vi "A 正面 处理函数2.vi"(7 "error in":errorcluster) -> (27 "error out":errorcluster)   [LabVIEW 2017]
uses:
  <vilib>/vision/Measure.llb/Edge Options.ctl
  <vilib>/vision/Measure.llb/Edge Polarity.ctl
  <vilib>/vision/Contour.llb/IMAQ Connect Range Setting.ctl
  <vilib>/vision/Contour.llb/IMAQ Contour Curve Extraction.ctl
  <vilib>/vision/Pattern Matching.llb/IMAQ Match Range Setting.ctl
  <vilib>/vision/NI_Vision_Development_Module.lvlib
panel:
  out "Image Out":T1(plugin-control)
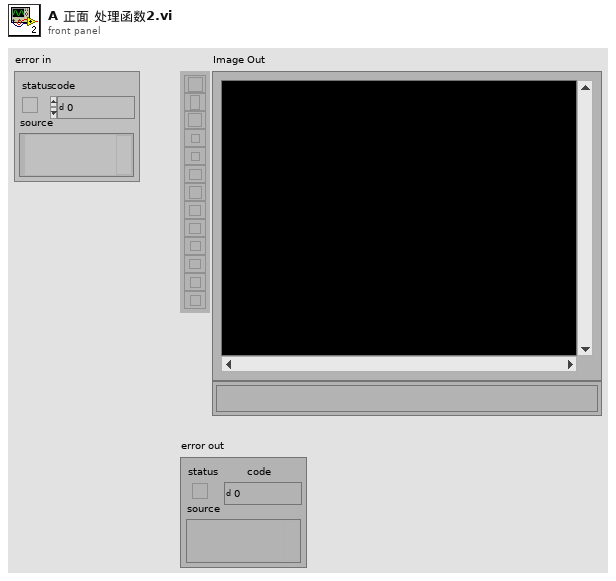
[diagram p1: front panel]
types:
  T1 = typedef "IMAQ Image.ctl" = refnum<image>
  T2 = typedef "IMAQ Match Range Setting.ctl" = cluster{"Match Constraints":u32, "Min":dbl, "Max":dbl}
  T3 = cluster{"Setup Data Item":u16, "Item Value":dbl}[]
  T4 = typedef "IMAQ Contour Curve Extraction.ctl" = cluster{"Extraction Mode":u32, "Edge Threshold":i32, "Edge Filter Size":u32, "Min Length":i32, "Search Step Size":i32, "Max Endpoint Gap":i32, "Subpixel":bool}
  T5 = cluster{"Rotation":bool, "Scale":bool, "Occlusion":bool}
  T6 = typedef "IMAQ Connect Range Setting.ctl" = cluster{"Match Constraints":u32, "Min":dbl, "Max":dbl}
  T7 = enum16{"Closest To Search Start", "Maximum Length", "Strongest Mean Gradient Change"}
  T8 = enum16{"Rect Left To Right", "Rect Right To Left", "Rect Top To Bottom", "Rect Bottom To Top", "Annulus Inner To Outer", "Annulus Outer To Inner", "Annulus Start Angle To End Angle", "Annulus End Angle To Start Angle"}
  T9 = cluster{"Overlay?":bool, "Color":u32, "Width":u32, "Maintain Width?":bool}
  T10 = cluster{"Global Rectangle":i32[], "Contours":cluster{"ID":enum32{"External", "Internal"}, "Type":u32, "Coordinates":i32[]}[]}
  T11 = cluster{"Origin":cluster{"X":sgl, "Y":sgl}, "Angle (deg)":sgl, "Axis Reference":u32}
  T12 = enum16{"Reset", "Update Coordinate System", "Get Coordinate System"}
  T13 = enum16{"Horizontal Motion", "Vertical Motion", "Horizontal and Vertical Motion", "Horizontal, Vertical and Angular Motion"}
  T14 = typedef "Edge Options.ctl" = cluster{"Edge Polarity":T15, "Kernel Size":u32, "Width":u32, "Minimum Edge Strength":sgl, "Interpolation Type":enum32{"Zero Order", "Bilinear", "Quadratic", "Cubic", "Bilinear Fixed"}, "Data Processing Method":enum32{"Average", "Median"}}
  T15 = typedef "Edge Polarity.ctl" = u32
  T16 = cluster{"Search  Direction":u32, "Edge Options":T14, "Show Search Area":bool, "Show Search Lines":bool, "Show Edges Found":bool, "Show Result":bool, "Search Area Color":u32, "Search Lines Color":u32, "Edge Locations Color":u32, "Result Color":u32, "Overlay Group Name":string}
  T17 = cluster{"Process":enum16{"Get First Edge", "Get First + Last Edge", "Get All Edges", "Get Best Edge"}, "Step Size":i32, "Max Pixel Radius":i32}
  T18 = typedef "Image Type" = u32
  T19 = cluster{"Center (Pixels)":cluster{"X":sgl, "Y":sgl}, "Radius (Pixels)":dbl, "Center (Real-World)":cluster{"X":sgl, "Y":sgl}, "Radius (Real-World)":dbl, "Roundness (Real-World)":dbl, "Average Strength":dbl, "Average SNR (dB)":dbl}
  T20 = typedef "IMAQ Coordinate System" = cluster{"Reference System":cluster{"Origin":cluster{"X":sgl, "Y":sgl}, "Angle (deg)":sgl, "Axis Reference":u32}, "Measurement System":cluster{"Origin":cluster{"X":sgl, "Y":sgl}, "Angle (deg)":sgl, "Axis Reference":u32}}
  T21 = typedef "ROI Descriptor" = cluster{"Global Rectangle":i32[], "Contours":cluster{"ID":enum32{"External", "Internal"}, "Type":u32, "Coordinates":i32[]}[]}
  T22 = cluster{"Target Point":cluster{"X":dbl, "Y":dbl}, "Template Point":cluster{"X":dbl, "Y":dbl}, "Distance":dbl}[]
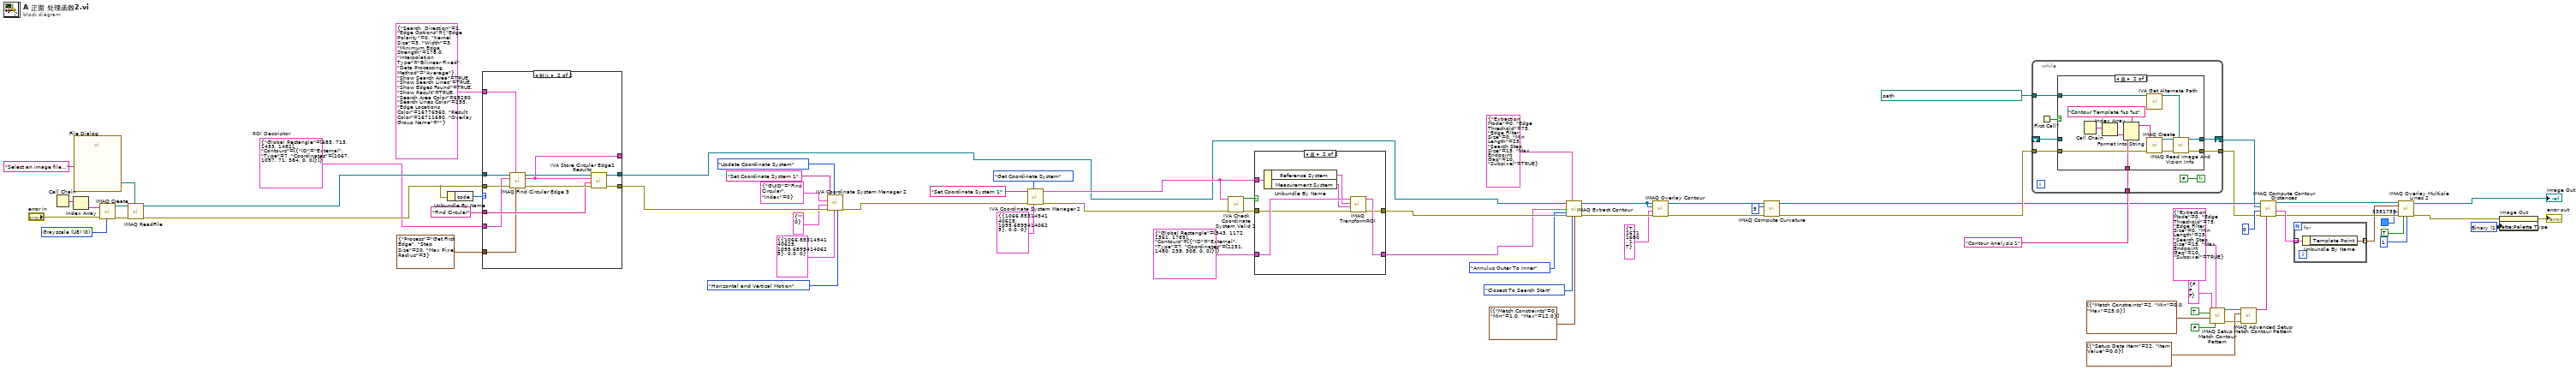
[diagram p0: block diagram]
diagram:
  w1 = u32 1 items=["Grayscale", "Binary", "Gradient", "Rainbow", "Temperature", "User Defined", "Binary 16 Bit", "Gradient 16 Bit", "Rainbow 16 Bit", "Temperature 16 Bit", "User Defined 16 Bit"] ("Palette Type")
  w59 = T10 {"Global Rectangle"=[683, 713, 1453, 1482], "Contours"=[{"ID"=enum."External", "Type"=7, "Coordinates"=[1067, 1097, 71, 384, 0, 0]}]}  # ROI Descriptor
  w63 = T18 0 items=["Grayscale (U8)", "Grayscale (I16)", "Grayscale (SGL)", "Complex (CSG)", "RGB (U32)", "HSL (U32)", "RGB (U64)", "Grayscale (U16)"] ("Image Type")
  n1 = Call Chain() -> (call chain=w67:string[])
  n2 = Index Array(array=w67) -> (element=w66:string)  [unwired: 1 in]
  n3 = call "File Dialog"("prompt"="Select an image file...") -> ("selected path"=w64:path)  [unwired: 6 in, 8 out]
  n4 = call "IMAQ Create"("Image Name"=w66, "Image Type"=w63, "error in (no error)"="error in") -> ("New Image"=w70:T1, "error out"=w69:errorcluster)  [unwired: 1 in, 1 out]
  n5 = call "IMAQ ReadFile"("File Path"=w64, "error in (no error)"=w69, "Image"=w70) -> ("error out"=w71:errorcluster, "Image Out"=w62:T1)  [unwired: 2 in, 5 out]
  n6 = Unbundle By Name(w71) -> ("code"=w58:i32)
  n7 = case "条件结构" shown="默认" w58 {
    tunnel: T16 {"Search  Direction"=1, "Edge Options"={"Edge Polarity"=0, "Kernel Size"=3, "Width"=3, "Minimum Edge Strength"=178.0, "Interpolation Type"=enum."Bilinear Fixed", "Data Processing Method"=enum."Average"}, "Show Search Area"=TRUE, "Show Search Lines"=TRUE, "Show Edges Found"=TRUE, "Show Result"=TRUE, "Search Area Color"=65280, "Search Lines Color"=255, "Edge Locations Color"=16776960, "Result Color"=16711680, "Overlay Group Name"=""} ("Options") -> [_ w73]
    tunnel: w62 -> [w72 w83]
    tunnel: w71 -> [_ w82]
    tunnel: [_ w80] -> w61
    tunnel: [w72 w78] -> w39
    tunnel: "Find Circular" ("Step Name") -> [_ w77]
    tunnel: w59 -> [_ w76]
    tunnel: T17 {"Process"=enum."Get First Edge", "Step Size"=20, "Max Pixel Radius"=3} ("Circle Fit Options") -> [_ w75]
    tunnel: [_ w74] -> _
    frame -1074396199, -1074396198 {
      # "Discard Coordinate System Error"
    }
    frame Default {
      n8 = call "IMAQ Find Circular Edge 3"("Circle Fit Options"=w75, "Options"=w73, "error in (no error)"=w82, "ROI Descriptor"=w76, "Image"=w83) -> ("error out"=w81:errorcluster, "Fitted Circle"=w74:T19, "Image Out"=w79:T1)  [unwired: 2 in, 2 out]
      n9 = call <vilib>:"IVA Store Circular Edge2 Results.vi"("error in (no error)"=w81, "Step Name"=w77, "Fitted Circle"=w74, "Image in"=w79) -> ("error out"=w80:errorcluster, "Image dup"=w78:T1)  [unwired: 2 in, 4 out]
    }
  }
  n10 = call <vilib>:"IVA Coordinate System Manager 2.vi"("Mode"=T13."Horizontal and Vertical Motion", "Reference System"=T11 {"Origin"={"X"=1066.8531, "Y"=1095.69}, "Angle (deg)"=0.0, "Axis Reference"=0}, "Function"=T12."Update Coordinate System", "error in (no error)"=w61, "Angle ID"=cluster{"GUID":string, "Index":i32} {"GUID"="", "Index"=0}, "Origin ID"=cluster{"GUID":string, "Index":i32} {"GUID"="Find Circular", "Index"=0}, "Coordinate System Name"="Set Coordinate System 1") -> ("error out"=w49:errorcluster)  [unwired: 4 out]
  n11 = call <vilib>:"IVA Coordinate System Manager 2.vi"("Reference System"=T11 {"Origin"={"X"=1066.8531, "Y"=1095.69}, "Angle (deg)"=0.0, "Axis Reference"=0}, "Function"=T12."Get Coordinate System", "error in (no error)"=w49, "Coordinate System Name"="Set Coordinate System 1") -> ("error out"=w46:errorcluster, "Coordinate System Out"=w42:T20)  [unwired: 3 in, 3 out]
  n12 = call <vilib>:"IVA Check Coordinate System Valid 2.vi"("error in (no error)"=w46, "Coordinate System"=w42) -> ("error out"=w40:errorcluster, "Valid?"=w41:bool)  [unwired: 8 out]
  n13 = case "条件结构" shown="真" w41 {
    tunnel: T10 {"Global Rectangle"=[943, 1172, 1561, 1789], "Contours"=[{"ID"=enum."External", "Type"=7, "Coordinates"=[1251, 1480, 238, 308, 0, 0]}]} ("ROI Descriptor") -> [w85 w92]
    tunnel: [w85 w89] -> w35
    tunnel: [w84 w88] -> w43
    tunnel: w42 -> [_ w87]
    tunnel: w40 -> [w84 w86]
    frame False {
    }
    frame True {
      n14 = Unbundle By Name(w87) -> ("Reference System"=w91:T11, "Measurement System"=w90:T11)
      n15 = call "IMAQ TransformROI"("error in (no error)"=w86, "New Reference"=w90, "Base Reference"=w91, "ROI Descriptor"=w92) -> ("error out"=w88:errorcluster, "ROI Descriptor out"=w89:T21)  [unwired: 6 out]
    }
  }
  n16 = call "IMAQ Extract Contour"("Source Image"=w39, "Curve Extraction"=T4 {"Extraction Mode"=0, "Edge Threshold"=75, "Edge Filter Size"=0, "Min Length"=25, "Search Step Size"=15, "Max Endpoint Gap"=10, "Subpixel"=TRUE}, "ROI Descriptor"=w35, "Search Direction"=T8."Annulus Outer To Inner", "error in (no error)"=w43, "Contour Selection"=T7."Closest To Search Start", "Curve Connection"=T6[] [{"Match Constraints"=0, "Min"=1.0, "Max"=12.0}]) -> ("Source Image Out"=w31:T1, "error out"=w38:errorcluster)  [unwired: 1 in, 6 out]
  n17 = call "IMAQ Overlay Contour"("error in (no error)"=w38, "Contour Points Settings"=T9 {"Overlay?"=TRUE, "Color"=16711680, "Width"=1, "Maintain Width?"=TRUE}, "Contour Image"=w31, "Image"=w31) -> ("error out"=w36:errorcluster, "Image Out"=w29:T1)  [unwired: 2 in, 4 out]
  n18 = call "IMAQ Compute Curvature"("error in (no error)"=w36, "Kernel Width"=u32 5, "Contour Image"=w29) -> ("error out"=w28:errorcluster, "Contour Image Out (dup)"=w23:T1)  [unwired: 1 in, 6 out]
  n19 = while "While循环" {
    tunnel: path "C:/Users/hedongpo/Desktop/吕亚/Temp3.png" ("Template File Path") -> [w100]
    tunnel: "Contour Analysis 1" ("Step Name") -> [w98]
    shift-right: [w96] -> w22
    shift-left: _ -> [w97]
    tunnel: w28 -> [w95]
    tunnel: [w94] -> w21
    stop <- FALSE continue-if-true
    n20 = First Call?() -> (First Call?: T/F=w99:bool)
    n21 = case "条件结构" shown="真" w99 {
      tunnel: [w102 w104] -> w96
      tunnel: w97 -> [w102 _]
      tunnel: [w101 w103] -> w94
      tunnel: w95 -> [w101 w109]
      tunnel: w100 -> [_ w114]
      tunnel: w98 -> [_ w105]
      frame False {
      }
      frame True {
        n22 = Call Chain() -> (call chain=w111:string[])
        n23 = Index Array(array=w111) -> (element=w110:string)  [unwired: 1 in]
        n24 = Format Into String(format string="Contour Template %s %s" ("Image Name"), w110, w105) -> (resulting string=w113:string)  [unwired: 2 in, 1 out]
        n25 = call <vilib>:"IVA Get Alternate Path.vi"("Path In"=w114) -> ("Path Out"=w106:path)  [unwired: 10 out]
        n26 = call "IMAQ Create"("Image Name"=w113, "error in (no error)"=w109) -> ("New Image"=w108:T1, "error out"=w107:errorcluster)  [unwired: 2 in, 1 out]
        n27 = call "IMAQ Read Image And Vision Info"("File Path"=w106, "error in (no error)"=w107, "Image"=w108) -> ("error out"=w103:errorcluster, "Image Out"=w104:T1)  [unwired: 1 in, 6 out]
      }
    }
  }
  n28 = call "IMAQ Setup Match Contour Pattern"("Use Learn Curve Extraction"=FALSE, "Curve Extraction"=T4 {"Extraction Mode"=0, "Edge Threshold"=75, "Edge Filter Size"=0, "Min Length"=25, "Search Step Size"=15, "Max Endpoint Gap"=10, "Subpixel"=TRUE} ("Curve Extraction 2"), "Range Settings"=T2[] [{"Match Constraints"=2, "Min"=0.0, "Max"=25.0}], "Subpixel Accuracy"=TRUE, "Match Mode"=T5 {"Rotation"=FALSE, "Scale"=FALSE, "Occlusion"=FALSE}) -> ("error out"=w4:errorcluster, "Match Contour Pattern Setup Data"=w8:string)  [unwired: 1 in, 4 out]
  n29 = call "IMAQ Advanced Setup Match Contour Pattern"("Match Contour Pattern Setup Data In"=w8, "Advanced Contour Match Options"=T3 [{"Setup Data Item"=22, "Item Value"=0.0}], "error in (no error)"=w4) -> ("Match Contour Pattern Setup Data Out"=w7:string)  [unwired: 7 out]
  n30 = call "IMAQ Compute Contour Distances"("Match Contour Pattern Setup Data"=w7, "error in (no error)"=w21, "Smoothing Kernel"=u32 0, "Template Contour Image"=w22, "Target Contour Image"=w23) -> ("error out"=w15:errorcluster, "Distances"=w17:T22, "Target Contour Image Out (dup)"=w16:T1)  [unwired: 4 out]
  n31 = for "For循环" {
    tunnel: w17 -> [w116] mode=indexing
    tunnel: [w115] -> w14 mode=indexing
    n32 = Unbundle By Name(w116) -> ("Template Point"=w115:cluster{"X":dbl, "Y":dbl})
  }
  n33 = call "IMAQ Overlay Multiple Lines 2"("Image"=w16, "Line End Points"=w14, "Color"=u32 3381759, "error in (no error)"=w15, "Maintain Width?"=TRUE, "Width"=u32 1) -> ("Image Out"=→"Image Out":T1, "error out"=w11:errorcluster)  [unwired: 2 in, 6 out]
  n34 = property on="Image Out" class="ImageControl"(error in=w11, "Palette:Palette Type"=w1) -> (error out=→"error out":errorcluster)  [unwired: 1 in, 1 out]
